vi "Polarizers.vi"(2 "Polarizers State":enum16{"OnBeam", "OffBeam"}(ring), 9 "error in (no error)":errorcluster) -> (6 "error out":errorcluster)   [LabVIEW 2009]
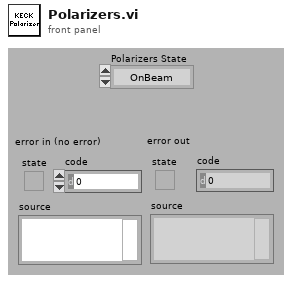
[diagram p1: front panel]
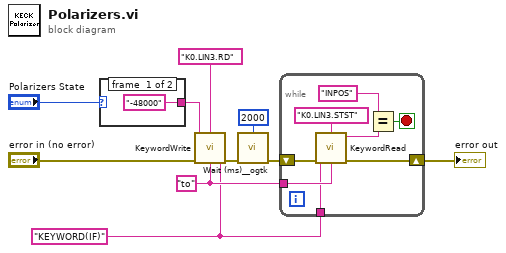
[diagram p0: block diagram]
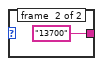
[diagram p2: hidden frame]
diagram:
  w1 = "KEYWORD(IF)" ("Crate")
  w2 = "to"
  n1 = case shown="\"OnBeam\"" "Polarizers State" {
    tunnel: ["-48000" "13700"] -> w7
    frame #0 {
    }
    frame #1 {
    }
  }
  n2 = call "KeywordWrite.vi"("Crate"=w1, "Keyword"="K0.LIN3.RD", "Value"=w7, "Service"=w2, "error in (no error)"="error in (no error)") -> ("error out"=w6:errorcluster)  [unwired: 4 out]
  n3 = call <userlib>:"Wait (ms)__ogtk.vi"("error in (no error)"=w6, "milliseconds to wait"=u32 2000) -> ("error out"=w4:errorcluster)  [unwired: 1 in, 8 out]
  n4 = while {
    shift-right: [w17] -> w3
    shift-left: w4 -> [w20]
    tunnel: w2 -> [w15]
    tunnel: w1 -> [w13]
    stop <- w18 stop-if-true
    n5 = call "KeywordRead.vi"("Keyword"="K0.LIN3.STST", "Crate"=w13, "Service"=w15, "error in (no error)"=w20) -> ("Value"=w14:string, "error out"=w17:errorcluster)  [unwired: 1 in, 3 out]
    n6 = Equal?(x="INPOS", y=w14) -> (x = y?=w18:bool)
  }
  "error out" <- w3
